vi "Configure Trigger IN.vi"(0 "VISA resource name":refnum<visa-resource-name>, 1 "Trigger In Source":u8(ring) items=["External", "Timer", "Button"], 3 "Ext Mod In Cond. Status":bool, 4 "Threshold (V)":dbl=1.0, 5 "error in (no error)":errorcluster, 6 "Timer Interval (s)":dbl=1.0, 7 "Trigger Slope":u8(ring) items=["Positive", "Negative", "Both"], 8 "Trigger In Cond. Status":bool, 10 "Ext Mod State":bool, 11 "Ext Mod Slope":u8(ring) items=["Positive", "Negative"], 12 "Ext Mod Threshold (V)":dbl min=-0.95 max=0.95, 13 "Selection Ext Mod":u8(ring) items=["Value", "Minimum", "Maximum", "Default"], 15 "Selection Timer Interval":u8(ring) items=["Value", "Minimum", "Maximum", "Default"], 18 "Trigger IN Impedance":u8(ring) items=["50 Ohm", "1K Ohm"]) -> (14 "VISA resource name out":refnum<visa-resource-name>, 19 "error out":errorcluster)   [LabVIEW 2020, in "Active Technologies AWG3000.lvlib"]
uses:
  Active Technologies AWG3000.lvlib
panel:
  in  "Selection Threshold Threshold":u8(ring) items=["Value", "Minimum", "Maximum", "Default"]
  # "Timer Reset Conditions"
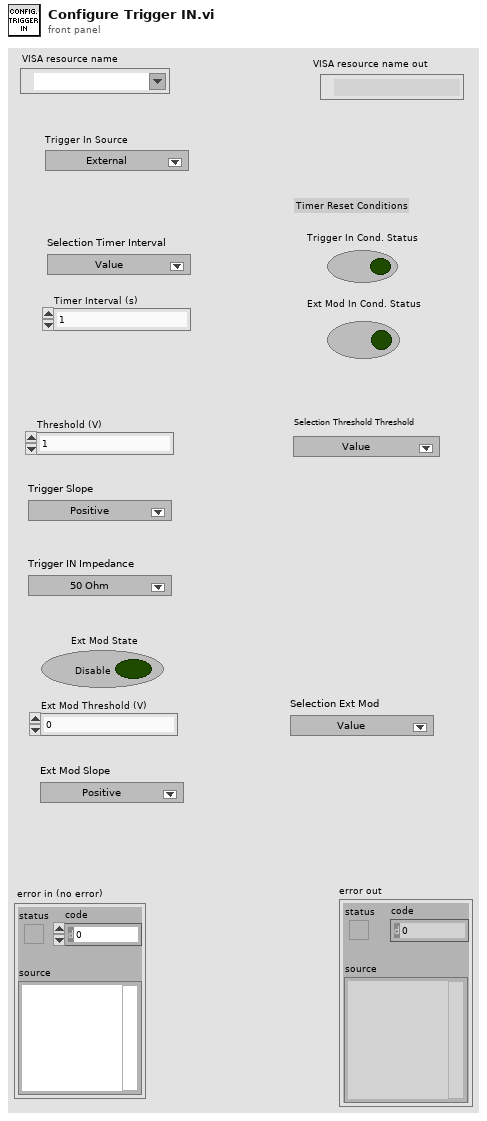
[diagram p1: front panel]
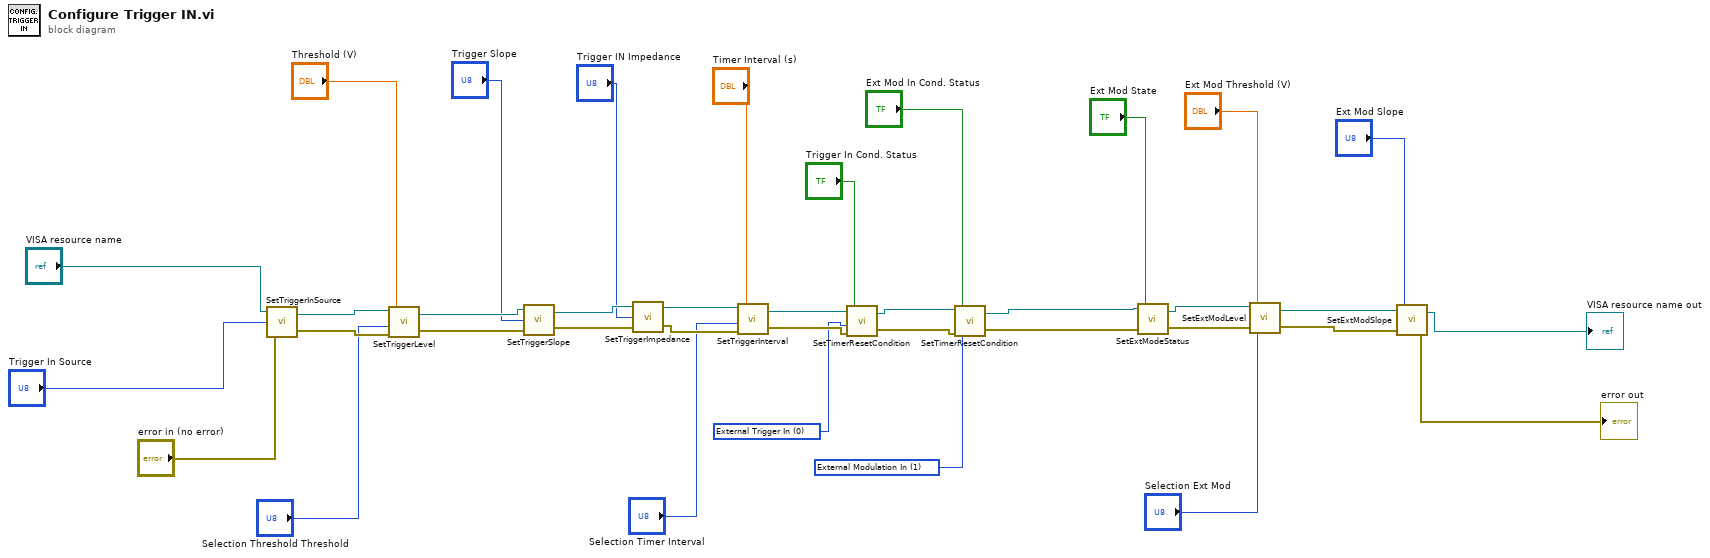
[diagram p0: block diagram]
diagram:
  w4 = u8 1 items=["External Trigger In", "External Modulation In"] ("Reset Timer Condition")
  w1 = u8 0 items=["External Trigger In", "External Modulation In"] ("Reset Timer Condition")
  n1 = call "SetTriggerInSource.vi"("error in (no error)"="error in (no error)", "Trigger In Source"="Trigger In Source", "VISA resource name"="VISA resource name") -> ("error out"=w33:errorcluster, "VISA resource name out"=w34:refnum<visa-resource-name>)
  n2 = call "SetTriggerLevel.vi"("error in (no error)"=w33, "Trigger In Selection"="Selection Threshold Threshold", "Trigger In Threshold (V)"="Threshold (V)", "VISA resource name"=w34) -> ("error out"=w30:errorcluster, "VISA resource name out"=w31:refnum<visa-resource-name>)
  n3 = call "SetTriggerSlope.vi"("error in (no error)"=w30, "Trigger In Slope"="Trigger Slope", "VISA resource name"=w31) -> ("error out"=w26:errorcluster, "VISA resource name out"=w27:refnum<visa-resource-name>)
  n4 = call "SetTriggerImpedance.vi"("error in (no error)"=w26, "Trigger IN Impedance"="Trigger IN Impedance", "VISA resource name"=w27) -> ("error out"=w23:errorcluster, "VISA resource name out"=w24:refnum<visa-resource-name>)
  n5 = call "SetTriggerInterval.vi"("error in (no error)"=w23, "Selection"="Selection Timer Interval", "Interval (s)"="Timer Interval (s)", "VISA resource name"=w24) -> ("error out"=w5:errorcluster, "VISA resource name out"=w8:refnum<visa-resource-name>)
  n6 = call "SetTimerResetCondition.vi"("error in (no error)"=w5, "Reset Timer Condition"=w1, "Timer Condition Status"="Trigger In Cond. Status", "VISA resource name"=w8) -> ("error out"=w6:errorcluster, "VISA resource name out"=w7:refnum<visa-resource-name>)
  n7 = call "SetTimerResetCondition.vi"("error in (no error)"=w6, "Reset Timer Condition"=w4, "Timer Condition Status"="Ext Mod In Cond. Status", "VISA resource name"=w7) -> ("error out"=w3:errorcluster, "VISA resource name out"=w2:refnum<visa-resource-name>)
  n8 = call "SetExtModeStatus.vi"("error in (no error)"=w3, "Ext Mod State"="Ext Mod State", "VISA resource name"=w2) -> ("error out"=w15:errorcluster, "VISA resource name out"=w16:refnum<visa-resource-name>)
  n9 = call "SetExtModLevel.vi"("error in (no error)"=w15, "Ext Mod Threshold (V)"="Ext Mod Threshold (V)", "Ext Mod Selection"="Selection Ext Mod", "VISA resource name"=w16) -> ("error out"=w13:errorcluster, "VISA resource name out"=w14:refnum<visa-resource-name>)
  n10 = call "SetExtModSlope.vi"("error in (no error)"=w13, "Ext Mod Slope"="Ext Mod Slope", "VISA resource name"=w14) -> ("error out"=→"error out":errorcluster, "VISA resource name out"=→"VISA resource name out":refnum<visa-resource-name>)
